vi "bee1v3.vi"() -> ()   [LabVIEW 2020]
uses:
  <vilib>/Instr/_visa.llb/VISA Flush IO Buffer Mask.ctl
  <vilib>/Instr/_visa.llb/VISA Configure Serial Port (Instr).vi
  <vilib>/Waveform/DWDTOps.llb/DWDT Boolean Array to Digital.vi
panel:
  in  "close":bool
  in  "start":bool
  in  "stop":bool
  in  "Tab Control":enum32{"Graph", " Config"}(tab)
  out "Digital Waveform Graph":digitalwaveform(graph)
  in  "FileName":string
  in  "VISA resource name":refnum<visa-resource-name>
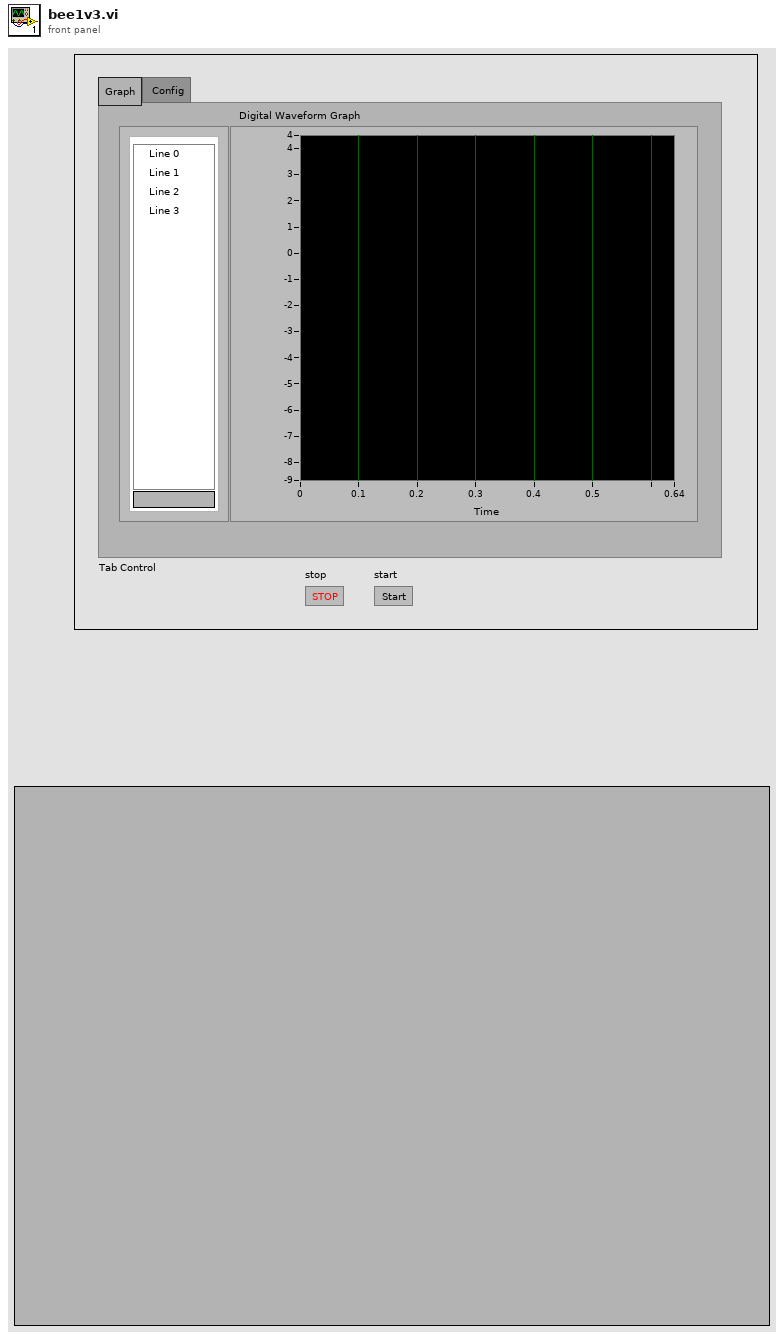
[diagram p1: front panel]
types:
  T1 = enum16{"open", "replace", "create", "open or create", "replace or create", "replace or create with confirmation"}
  T2 = typedef "VISA Flush IO Buffer Mask.ctl" = u16
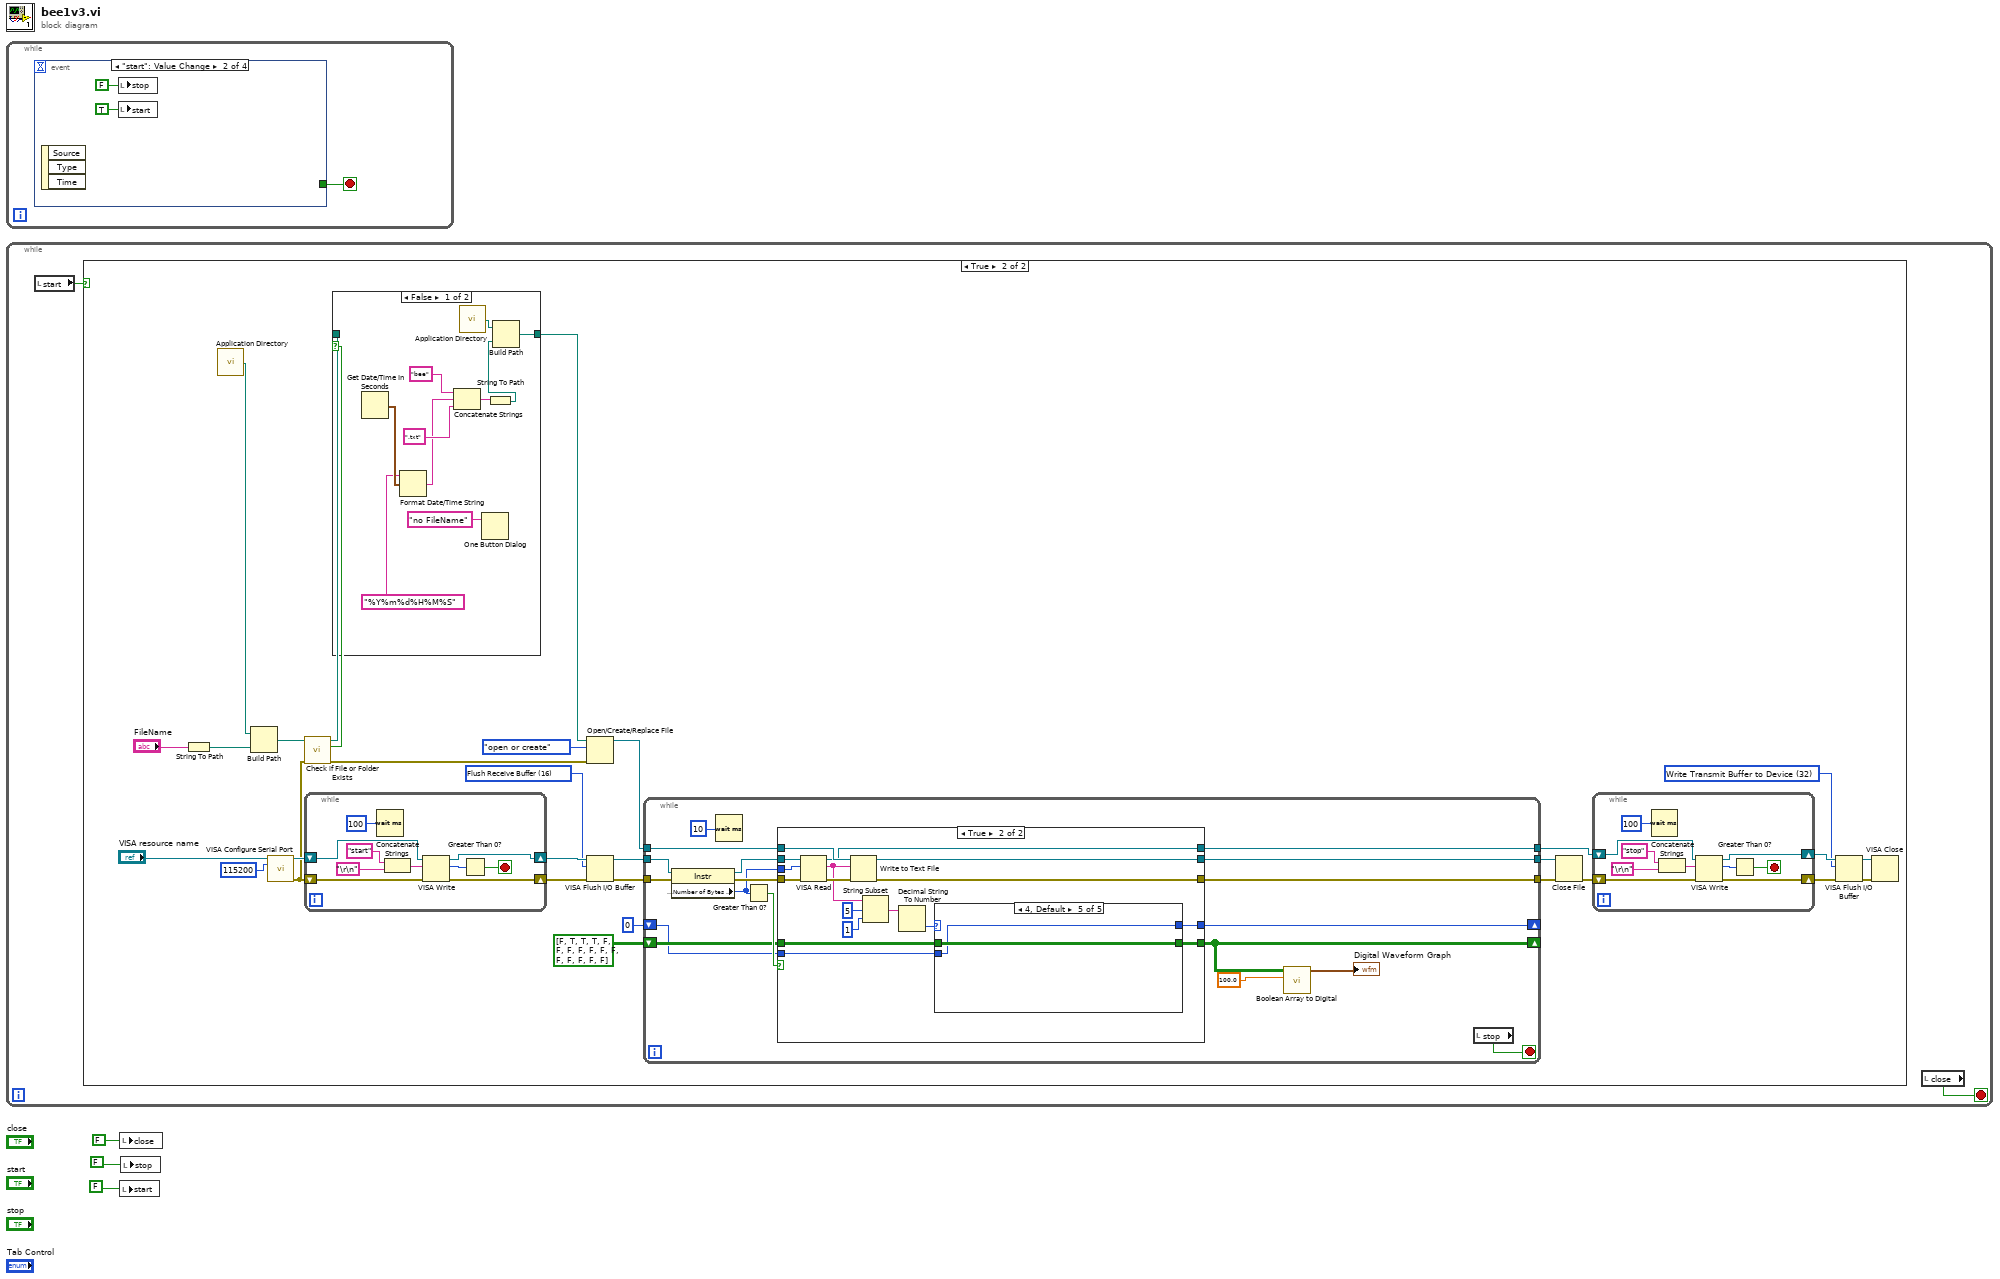
[diagram p0: block diagram]
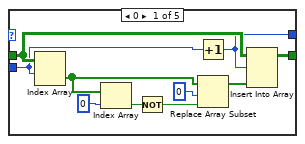
[diagram p5: hidden frame]
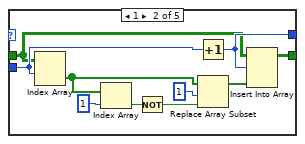
[diagram p6: hidden frame]
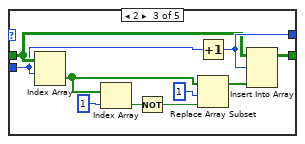
[diagram p7: hidden frame]
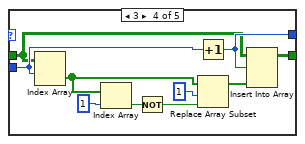
[diagram p8: hidden frame]
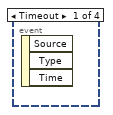
[diagram p9: hidden frame]
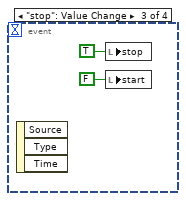
[diagram p10: hidden frame]
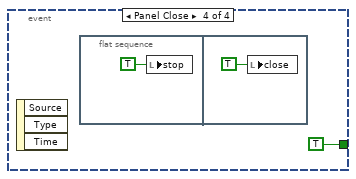
[diagram p11: hidden frame]
diagram:
  n1 = while {
    stop <- w4 stop-if-true
    n2 = event shown="[1] \"start\": Value Change" {
      selector: _ -> [_ _ _ _]
      dyn-events: _ -> [_ _ _ _]
      timeout: _ -> [_ _ _ _]
      tunnel: [_ _ _ TRUE] -> w4
      event Timeout {
        n3 = event-data() -> ()  [unwired: 1 in, 3 out]
      }
      event "start": Value Change {
        n4 = event-data() -> ()  [unwired: 1 in, 3 out]
        n5 = local write "stop"(FALSE) -> ()
        n6 = local write "start"(TRUE) -> ()
      }
      event "stop": Value Change {
        n7 = event-data() -> ()  [unwired: 1 in, 3 out]
        n8 = local write "stop"(TRUE) -> ()
        n9 = local write "start"(FALSE) -> ()
      }
      event Panel Close {
        n10 = event-data() -> ()  [unwired: 1 in, 3 out]
        n11 = flat-sequence {
          frame #0 {
            n12 = local write "stop"(TRUE) -> ()
          }
          frame #1 {
            n13 = local write "close"(TRUE) -> ()
          }
        }
      }
    }
  }
  n14 = while {
    stop <- w12 stop-if-true
    n15 = local read "start"() -> (w13:bool)
    n16 = case shown="True" w13 {
      frame False {
      }
      frame True {
        w25 = T2 32 items=["Flush Receive Buffer"=16, "Write Transmit Buffer to Device"=32, "Flush Receive Buffer (No I/O)"=64, "Flush Transmit Buffer"=128] ("Mask")
        w30 = T2 16 items=["Flush Receive Buffer"=16, "Write Transmit Buffer to Device"=32, "Flush Receive Buffer (No I/O)"=64, "Flush Transmit Buffer"=128] ("Mask")
        n17 = String To Path(string="FileName") -> (path=w20:path)
        n18 = call <vilib>:"Application Directory.vi"() -> ("Application Directory"=w40:path)
        n19 = Build Path(base path=w40, name or relative path=w20) -> (appended path=w17:path)
        n20 = call-poly "VISA Configure Serial Port"("VISA resource name"="VISA resource name", "baud rate (9600)"=u32 115200) -> ("VISA resource name out"=w38:refnum<visa-resource-name>, "error out"=w19:errorcluster)  [unwired: 12 in]
        n21 = call <vilib>:"Check if File or Folder Exists.vi"("error in (no error)"=w19, "path"=w17) -> ("error out"=w18:errorcluster, "file or folder exists?"=w16:bool, "dup path"=w15:path)  [unwired: 7 in]
        n22 = while {
          shift-right: [w66] -> w34
          shift-left: w38 -> [w74]
          shift-right: [w65] -> w33
          shift-left: w19 -> [w73]
          stop <- w72 stop-if-true
          n23 = Wait (ms)(milliseconds to wait=u32 100) -> ()  [unwired: 1 out]
          n24 = Concatenate Strings("start" ("write buffer"), "\r\n") -> (w67:string)
          n25 = VISA Write(VISA resource name=w74, write buffer=w67, error in (no error)=w73) -> (VISA resource name out=w66:refnum<visa-resource-name>, return count=w71:u32, error out=w65:errorcluster)
          n26 = Greater Than 0?(x=w71) -> (x > 0?=w72:bool)
        }
        n27 = case shown="False" w16 {
          tunnel: w15 -> [_ w54]
          tunnel: [w52 w54] -> w14
          frame False {
            n28 = Get Date/Time In Seconds() -> (seconds since 1Jan1904=w47:timestamp)
            n29 = Format Date/Time String(time format string (%c)="%Y%m%d%H%M%S", seconds (now)=w47) -> (date/time string=w44:string)  [unwired: 1 in]
            n30 = Concatenate Strings("bee" ("string"), w44, ".txt" ("string")) -> (w50:string)
            n31 = call <vilib>:"Application Directory.vi"() -> ("Application Directory"=w53:path)
            n32 = One Button Dialog(message="no FileName") -> ()  [unwired: 1 in, 1 out]
            n33 = String To Path(string=w50) -> (path=w49:path)
            n34 = Build Path(base path=w53, name or relative path=w49) -> (appended path=w52:path)
          }
          frame True {
          }
        }
        n35 = Open/Create/Replace File(file path (use dialog)=w14, error in=w18, operation (0:open)=T1."open or create") -> (refnum out=w41:refnum<file>)  [unwired: 3 in, 2 out]
        n36 = VISA Flush I/O Buffer(VISA resource name=w34, mask (16)=w30, error in (no error)=w33) -> (VISA resource name out=w32:refnum<visa-resource-name>, error out=w31:errorcluster)
        n37 = while {
          tunnel: w32 -> [w92]
          tunnel: w31 -> [w82]
          tunnel: w41 -> [w87]
          tunnel: [w86] -> w23
          tunnel: [w85] -> w24
          tunnel: [w84] -> w37
          shift-right: [w77] -> _
          shift-left: bool[][] [[FALSE, TRUE, TRUE, TRUE], [FALSE, FALSE, FALSE, FALSE], [FALSE, FALSE, FALSE, FALSE], [FALSE, FALSE, FALSE, FALSE]] -> [w80]
          shift-right: [w78] -> _
          shift-left: 0 -> [w79]
          stop <- w76 stop-if-true
          n38 = property class="Instr"(reference=w92, error in=w82) -> (reference out=w90:refnum<visa-resource-name>, error out=w91:errorcluster, "Serial Settings:Number of Bytes at Serial Port"=w88:u32)
          n39 = Wait (ms)(milliseconds to wait=10 ("timeout in ms (-1)")) -> ()  [unwired: 1 out]
          n40 = Greater Than 0?(x=w88) -> (x > 0?=w89:bool)
          n41 = case shown="True" w89 {
            tunnel: w91 -> [w96 w114]
            tunnel: w90 -> [w95 w113]
            tunnel: w88 -> [_ w112]
            tunnel: w87 -> [w97 w111]
            tunnel: [w97 w109] -> w86
            tunnel: [w96 w108] -> w85
            tunnel: [w95 w107] -> w84
            tunnel: [w94 w101] -> w77
            tunnel: w80 -> [w94 w100]
            tunnel: w79 -> [w93 w99]
            tunnel: [w93 w98] -> w78
            frame False {
            }
            frame True {
              n42 = VISA Read(VISA resource name=w113, byte count=w112, error in (no error)=w114) -> (VISA resource name out=w107:refnum<visa-resource-name>, read buffer=w102:string, error out=w110:errorcluster)  [unwired: 1 out]
              n43 = Write to Text File(file (use dialog)=w111, text=w102, error in=w110) -> (refnum out=w109:refnum<file>, error out=w108:errorcluster)  [unwired: 1 in, 1 out]
              n44 = String Subset(string=w102, offset (0)=5, length (rest)=1 ("length (rest)")) -> (substring=w104:string)
              n45 = Decimal String To Number(string=w104) -> (number=w103:i32)  [unwired: 2 in, 1 out]
              n46 = case shown="4, Default" w103 {
                tunnel: [w117 w134 w137 w148 w156] -> w101
                tunnel: w100 -> [w118 w131 w136 w145 w156]
                tunnel: w99 -> [w115 w133 w135 w146 w155]
                tunnel: [w116 w132 w138 w147 w155] -> w98
                frame 0 {
                  n47 = Index Array(array=w118, index (row)=w115) -> (element=w121:bool[])  [unwired: 1 in]
                  n48 = Index Array(array=w121, index=0) -> (element=w124:bool)
                  n49 = Not(x=w124) -> (.not. x?=w123:bool)
                  n50 = Increment(x=w115) -> (x+1=w116:i32)
                  n51 = Replace Array Subset(array=w121, new element=w123, index=0) -> (w122:bool[])
                  n52 = Insert Into Array(array=w118, index (row)=w116, new element=w122) -> (w117:bool[][])  [unwired: 1 in]
                }
                frame 1 {
                  n53 = Index Array(array=w131, index (row)=w133) -> (element=w129:bool[])  [unwired: 1 in]
                  n54 = Index Array(array=w129, index=1) -> (element=w125:bool)
                  n55 = Not(x=w125) -> (.not. x?=w126:bool)
                  n56 = Increment(x=w133) -> (x+1=w132:i32)
                  n57 = Replace Array Subset(array=w129, new element=w126, index=1) -> (w127:bool[])
                  n58 = Insert Into Array(array=w131, index (row)=w132, new element=w127) -> (w134:bool[][])  [unwired: 1 in]
                }
                frame 2 {
                  n59 = Index Array(array=w136, index (row)=w135) -> (element=w141:bool[])  [unwired: 1 in]
                  n60 = Index Array(array=w141, index=1) -> (element=w144:bool)
                  n61 = Not(x=w144) -> (.not. x?=w143:bool)
                  n62 = Increment(x=w135) -> (x+1=w138:i32)
                  n63 = Replace Array Subset(array=w141, new element=w143, index=1) -> (w142:bool[])
                  n64 = Insert Into Array(array=w136, index (row)=w138, new element=w142) -> (w137:bool[][])  [unwired: 1 in]
                }
                frame 3 {
                  n65 = Index Array(array=w145, index (row)=w146) -> (element=w153:bool[])  [unwired: 1 in]
                  n66 = Index Array(array=w153, index=1) -> (element=w149:bool)
                  n67 = Not(x=w149) -> (.not. x?=w150:bool)
                  n68 = Increment(x=w146) -> (x+1=w147:i32)
                  n69 = Replace Array Subset(array=w153, new element=w150, index=1) -> (w151:bool[])
                  n70 = Insert Into Array(array=w145, index (row)=w147, new element=w151) -> (w148:bool[][])  [unwired: 1 in]
                }
                frame 4, Default {
                }
              }
            }
          }
          n71 = call-poly <vilib>:"Boolean Array to Digital.vi"("sample rate"=100.0, "boolean array"=w77) -> ("digital waveform"=→"Digital Waveform Graph":digitalwaveform)  [unwired: 8 in, 1 out]
          n72 = local read "stop"() -> (w76:bool)
        }
        n73 = Close File(refnum=w23, error in=w24) -> (error out=w22:errorcluster)  [unwired: 1 out]
        n74 = while {
          shift-right: [w59] -> w28
          shift-left: w22 -> [w58]
          shift-right: [w60] -> w29
          shift-left: w37 -> [w64]
          stop <- w56 stop-if-true
          n75 = Wait (ms)(milliseconds to wait=u32 100) -> ()  [unwired: 1 out]
          n76 = Concatenate Strings("stop" ("write buffer"), "\r\n") -> (w61:string)
          n77 = VISA Write(VISA resource name=w64, write buffer=w61, error in (no error)=w58) -> (VISA resource name out=w60:refnum<visa-resource-name>, return count=w57:u32, error out=w59:errorcluster)
          n78 = Greater Than 0?(x=w57) -> (x > 0?=w56:bool)
        }
        n79 = VISA Flush I/O Buffer(VISA resource name=w29, mask (16)=w25, error in (no error)=w28) -> (VISA resource name out=w26:refnum<visa-resource-name>, error out=w27:errorcluster)
        n80 = VISA Close(VISA resource name=w26, error in (no error)=w27) -> ()  [unwired: 1 out]
      }
    }
    n81 = local read "close"() -> (w12:bool)
  }
  n82 = local write "close"(FALSE) -> ()
  n83 = local write "start"(FALSE) -> ()
  n84 = local write "stop"(FALSE) -> ()
